vi "Read Values from File.vi"(8 "Error at input":errorcluster, 11 "File Path":path) -> (0 "Error at reading spreadsheet":errorcluster, 1 "Left Spindle Difference":dbl, 2 "Center Spindle Difference":dbl, 3 "Right Spindle Difference":dbl)   [LabVIEW 2016]
uses:
  <vilib>/Utility/file.llb/Read Delimited Spreadsheet (string).vi
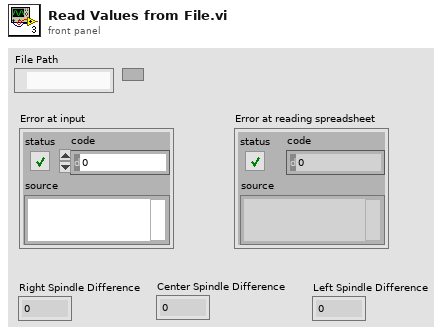
[diagram p1: front panel]
types:
  T1 = cluster{"all rows[0]":string, "all rows[1]":string, "all rows[2]":string, "all rows[3]":string, "all rows[4]":string, "all rows[5]":string, "all rows[6]":string, "all rows[7]":string, "all rows[8]":string}
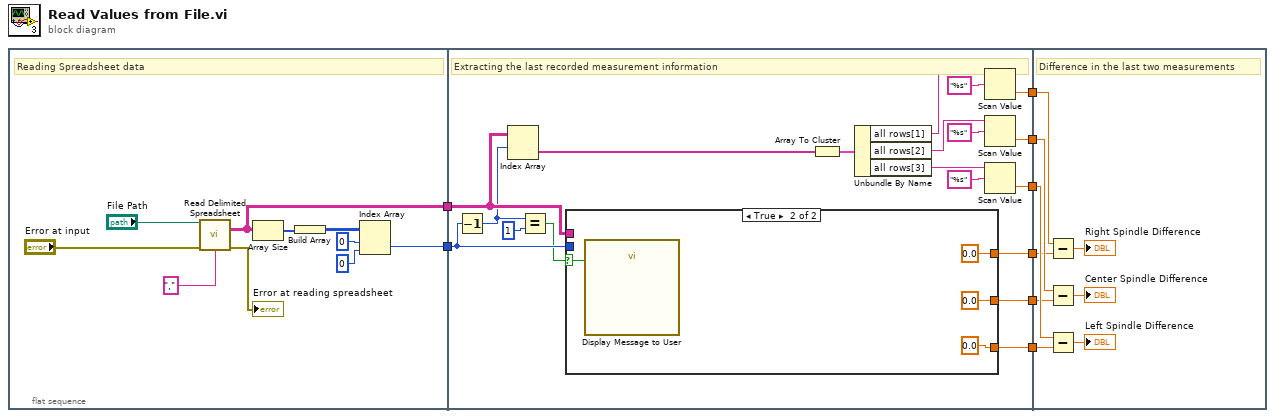
[diagram p0: block diagram]
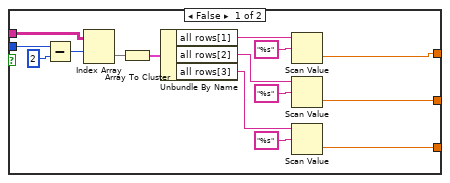
[diagram p2: hidden frame]
diagram:
  n1 = flat-sequence {
    tunnel: [w10] -> w8
    tunnel: [w9] -> w7
    tunnel: w8 -> [w30]
    tunnel: w7 -> [w22]
    tunnel: [w28] -> w6
    tunnel: [w27] -> w5
    tunnel: [w26] -> w4
    tunnel: [w25] -> w3
    tunnel: [w24] -> w2
    tunnel: [w23] -> w1
    tunnel: w6 -> [w65]
    tunnel: w5 -> [w61]
    tunnel: w4 -> [w60]
    tunnel: w3 -> [w59]
    tunnel: w2 -> [w58]
    tunnel: w1 -> [w57]
    frame #0 {
      # "Reading Spreadsheet data"
      n2 = call-poly <vilib>:"Read Delimited Spreadsheet.vi"("file path (dialog if empty)"="File Path", "error in (no error)"="Error at input", "delimiter (\\t)"="," ("delimiter (\\t)")) -> ("all rows"=w10:string[][], "error out"=→"Error at reading spreadsheet":errorcluster)  [unwired: 7 in, 4 out]
      n3 = Array Size(array=w10) -> (size(s)=w16:i32[])
      n4 = Build Array(w16) -> (w15:i32[][])
      n5 = Index Array(array=w15, index (row)=0, index (col)=0 ("disabled index (col)")) -> (element=w9:i32)
    }
    frame #1 {
      # "Extracting the last recorded measurement information"
      n6 = Decrement(x=w22) -> (x-1=w21:i32)
      n7 = Index Array(array=w30, index (row)=w21) -> (element=w29:string[])  [unwired: 1 in]
      n8 = Equal?(x=w21, y=1) -> (x = y?=w19:bool)
      n9 = case shown="True" w19 {
        selector: w19 -> [_ w53]
        tunnel: w30 -> [w46 _]
        tunnel: [w41 0.0] -> w25
        tunnel: [w40 0.0] -> w24
        tunnel: [w39 0.0] -> w23
        tunnel: w22 -> [w38 _]
        frame False {
          n10 = Subtract(x=w38, y=2) -> (x-y=w52:i32)
          n11 = Index Array(array=w46, index (row)=w52) -> (element=w45:string[])  [unwired: 1 in]
          n12 = Array To Cluster(array=w45) -> (cluster=w51:T1)
          n13 = Unbundle By Name(w51) -> ("all rows[1]"=w44:string, "all rows[2]"=w43:string, "all rows[3]"=w42:string)
          n14 = Scan Value(string=w44, format string="%s") -> (value=w41:dbl)  [unwired: 1 in, 1 out]
          n15 = Scan Value(string=w43, format string="%s") -> (value=w40:dbl)  [unwired: 1 in, 1 out]
          n16 = Scan Value(string=w42, format string="%s") -> (value=w39:dbl)  [unwired: 1 in, 1 out]
        }
        frame True {
          n17 = call "Display Message to User"("Enable"=w53) -> ()  [unwired: 9 in, 2 out]
        }
      }
      n18 = Array To Cluster(array=w29) -> (cluster=w31:T1)
      n19 = Unbundle By Name(w31) -> ("all rows[1]"=w32:string, "all rows[2]"=w35:string, "all rows[3]"=w37:string)
      n20 = Scan Value(string=w32, format string="%s") -> (value=w28:dbl)  [unwired: 1 in, 1 out]
      n21 = Scan Value(string=w35, format string="%s") -> (value=w27:dbl)  [unwired: 1 in, 1 out]
      n22 = Scan Value(string=w37, format string="%s") -> (value=w26:dbl)  [unwired: 1 in, 1 out]
    }
    frame #2 {
      # "Difference in the last two measurements"
      n23 = Subtract(x=w65, y=w59) -> (x-y=→"Right Spindle Difference":dbl)
      n24 = Subtract(x=w61, y=w58) -> (x-y=→"Center Spindle Difference":dbl)
      n25 = Subtract(x=w60, y=w57) -> (x-y=→"Left Spindle Difference":dbl)
    }
  }
